vi "AreaDeUnTriangulo.vi"() -> ()   [LabVIEW 2020]
panel:
  out "Numeric":dbl
  in  "ALTURA":dbl
  in  "BASE":dbl
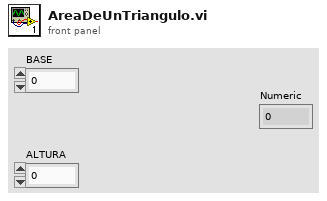
[diagram p1: front panel]
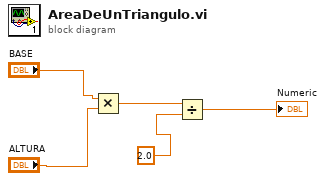
[diagram p0: block diagram]
diagram:
  n1 = Multiply(x="BASE", y="ALTURA") -> (x*y=w3:dbl)
  n2 = Divide(x=w3, y=2.0) -> (x/y=→"Numeric":dbl)
